vi "Tool Q LEIN solonoid valve task.vi"(0 "Main Controller ID":u8=42, 1 "Retry on err (F)":bool, 2 "Solonoid ID":u8=16, 5 "current limit(0.2A)":dbl, 7 "outpuyt channel":u8, 9 "time (50 ms)":u16, 11 "error in (no error)":errorcluster) -> (4 "LEIN custom reply Q":T1, 15 "error out":errorcluster)   [LabVIEW 2011]
uses:
  LEINmaster/Defenitions/LEIN custom reply Q.ctl
  LEINmaster/Defenitions/LEIN Reply Holder.ctl
  LEINmaster/Defenitions/LEIN CMD Cluster.ctl
  LEINmaster/Defenitions/LEIN CMD List.ctl
  LEINmaster/Defenitions/LEIN Structure variations.ctl
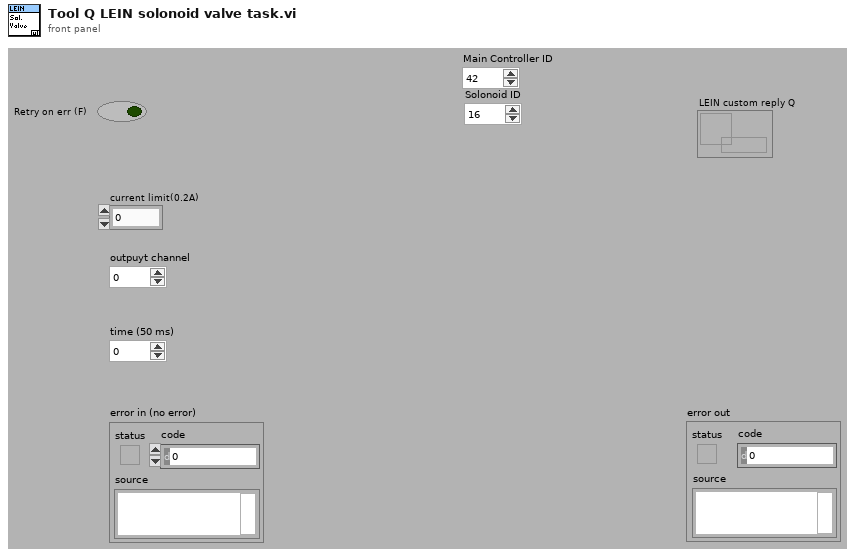
[diagram p1: front panel]
types:
  T1 = typedef "LEIN custom reply Q.ctl" = refnum<queue>
  T2 = typedef "LEIN Structure variations.ctl" = enum16{"LEIN08", "LEIN31", "LEIN63"}
  T3 = enum16{"big-endian, network order", "native, host order", "little-endian"}
  T4 = typedef "LEIN CMD Cluster.ctl" = cluster{"SID":u8, "ANF":bool, "CMD":T5, "DATA":u8[]}
  T5 = typedef "LEIN CMD List.ctl" = enum8{"ACTI", "TASK", "RES0", "STAT", "RES1", "RES2", "RES3", "USER"}
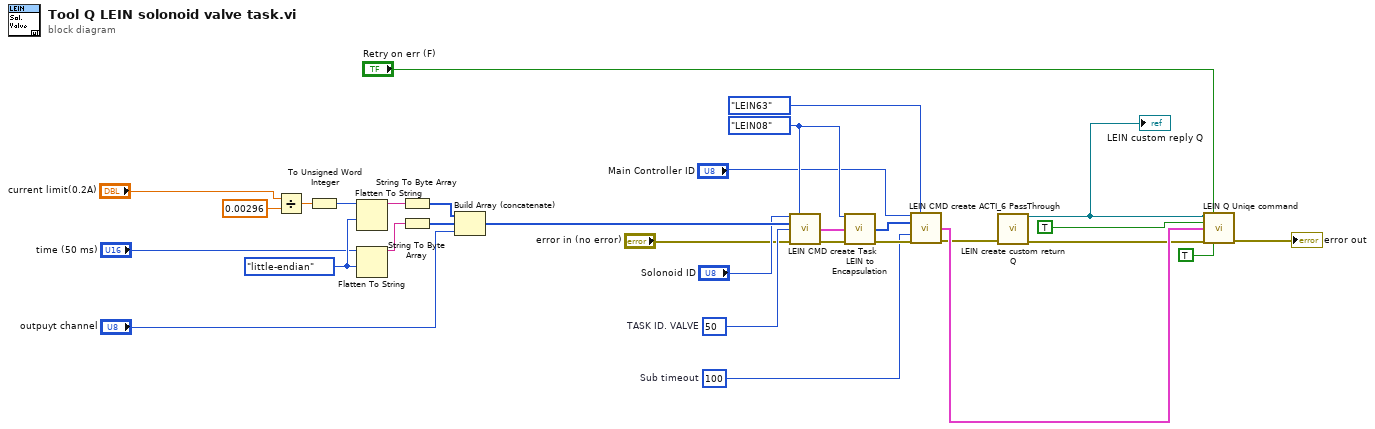
[diagram p0: block diagram]
diagram:
  w16 = u16 100  # Sub timeout
  w13 = u8 50  # TASK ID. VALVE
  w12 = LEIN_Structure_variations."LEIN08" ("LEIN Variation")
  w25 = T3."little-endian" ("byte order (0:big-endian, network order)")
  n1 = Divide(x="current limit(0.2A)", y=0.00296 ("x")) -> (x/y=w30:dbl)
  n2 = To Unsigned Word Integer(number=w30) -> (unsigned 16bit integer=w28:u16)
  n3 = Flatten To String(anything=w28, byte order (0:big-endian, network order)=w25) -> (data string=w27:string)  [unwired: 2 in, 2 out]
  n4 = Flatten To String(anything="time (50 ms)", byte order (0:big-endian, network order)=w25) -> (data string=w23:string)  [unwired: 2 in, 2 out]
  n5 = String To Byte Array(string=w27) -> (unsigned byte array=w26:u8[])
  n6 = String To Byte Array(string=w23) -> (unsigned byte array=w22:u8[])
  n7 = Build Array (concatenate)(w26, w22, "outpuyt channel") -> (w11:u8[])
  n8 = call "LEIN CMD create Task.vi"("SID"="Solonoid ID", "LEIN Variation"=w12, "Data"=w11, "TASK ID"=w13, "error in (no error)"="error in (no error)") -> ("CMD"=w14:T4, "error out"=w15:errorcluster)  [unwired: 9 in]
  n9 = call "LEIN to Encapsulation.vi"("LEIN Variation"=w12, "CMD"=w14, "error in (no error)"=w15) -> ("Data and header"=w17:u8[], "error out"=w18:errorcluster)  [unwired: 8 in, 3 out]
  n10 = call "LEIN CMD create ACTI_6 PassThrough.vi"("SID"="Main Controller ID", "LEIN Variation"=LEIN_Structure_variations."LEIN63", "LEIN ecapsulated data (header and data)"=w17, "Sub Timeout (ms)"=w16, "error in (no error)"=w18) -> ("CMD"=w5:T4, "error out"=w4:errorcluster)  [unwired: 9 in]
  n11 = call "LEIN create custom return Q.vi"("error in (no error)"=w4) -> ("LEIN custom reply Q"=w2:T1, "error out"=w3:errorcluster)  [unwired: 13 in]
  "LEIN custom reply Q" <- w2
  n12 = call "LEIN Q Uniqe command.vi"("LEIN custom reply Q"=w2, "Retry on err (F)"="Retry on err (F)", "Custom Q(F)"=TRUE, "CMD"=w5, "error in"=w3, "priority(F)"=TRUE) -> ("error out"=→"error out":errorcluster)  [unwired: 9 in]
